vi "Fetch Column name.vi"(8 "error in (no error)":errorcluster, 10 "Table name":string, 11 "Access in":refnum<class "Access.lvclass">) -> (0 "error out":errorcluster, 2 "columns":string[](array[string]), 3 "Access out":refnum<class "Access.lvclass">)   [LabVIEW 2021, in "Database.lvlib" / "Access.lvclass"]
uses:
  Access.lvclass
  Access.lvclass/Access.ctl
  <vilib>/addons/database/NI_Database_API.lvlib
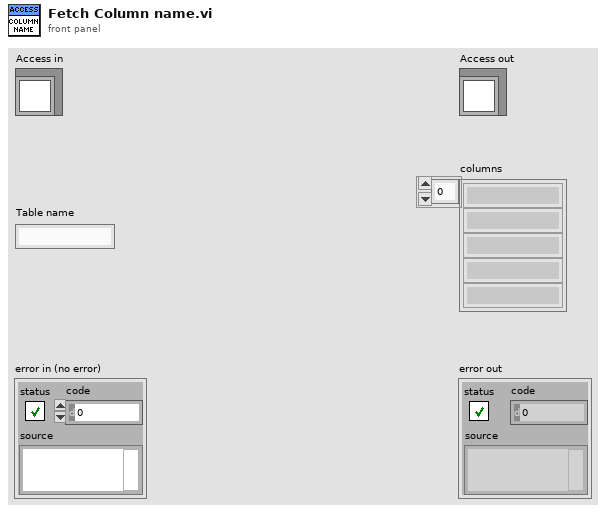
[diagram p1: front panel]
types:
  T1 = typedef "NI_Database_API.lvlib/Conn ObjectReference.ctl" = refnum<k1>
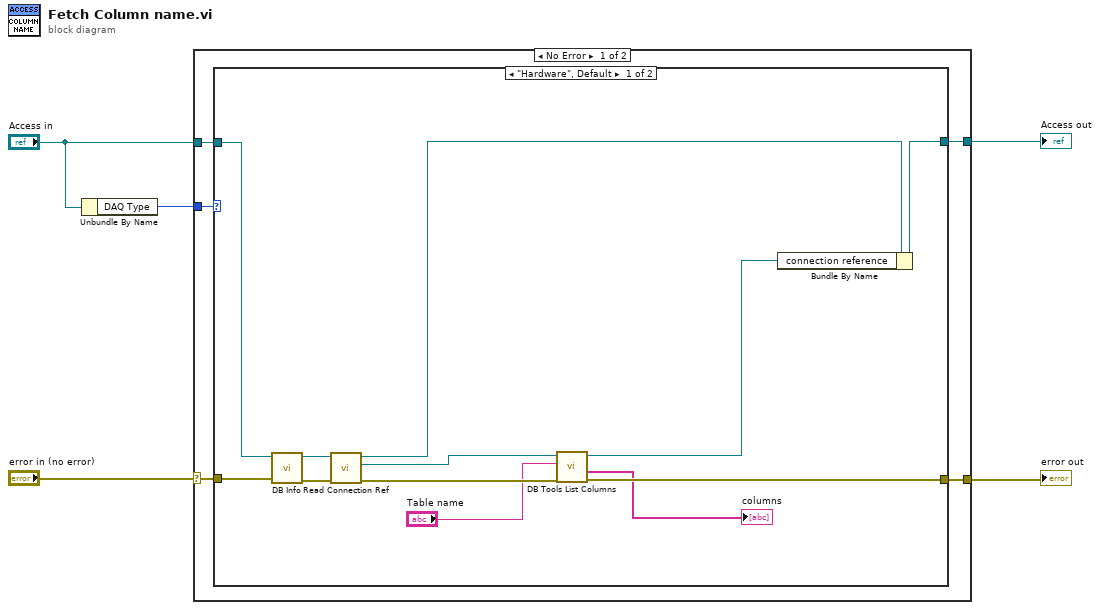
[diagram p0: block diagram]
diagram:
  n1 = Unbundle By Name("Access in") -> ("DAQ Type"=w3:enum16{"Hardware", "Simulation"})
  n2 = case shown="No Error" "error in (no error)" {
    selector: "error in (no error)" -> [w8 w25]
    tunnel: "Access in" -> [w9 w26]
    tunnel: w3 -> [w10 _]
    tunnel: [w7 w26] -> w2
    tunnel: [w6 w25] -> w1
    frame No Error {
      n3 = case shown="\"Hardware\", Default" w10 {
        tunnel: w9 -> [w15 w23]
        tunnel: w8 -> [w22 w24]
        tunnel: [w17 w23] -> w7
        tunnel: [w13 w24] -> w6
        frame "Hardware", Default {
          n4 = call-dynamic "DB Info.vi"("error in (no error)"=w22, "Access in"=w15) -> ("error out"=w20:errorcluster, "Access out"=w21:refnum<class "Access.lvclass">)  [unwired: 6 in, 2 out]
          n5 = call-dynamic "Read Connection Ref.vi"("error in (no error)"=w20, "Access in"=w21) -> ("error out"=w18:errorcluster, "connection reference"=w19:T1, "Access out"=w14:refnum<class "Access.lvclass">)  [unwired: 7 in]
          n6 = call <vilib>:"DB Tools List Columns.vi"("error in (no error)"=w18, "table"="Table name", "connection reference"=w19) -> ("error out"=w13:errorcluster, "columns"=→"columns":string[], "connection reference out"=w16:T1)  [unwired: 1 in, 1 out]
          n7 = Bundle By Name(cluster=w14, "connection reference"=w16) -> (w17:refnum<class "Access.lvclass">)
        }
        frame "Simulation" {
        }
      }
    }
    frame Error {
    }
  }
  "error out" <- w1
  "Access out" <- w2
